vi "Create Private Data for Get Connections Tests.vi"(9 "session":variant, 10 "channel mappings":T1[](array[typedef]), 11 "instrument_type_id":string) -> (3 "data":T2)   [LabVIEW 2020, in "MeasurementServerTests.lvlib"]
uses:
  MeasurementServerTests.lvlib
  Runtime/MeasurementLink Session Management/Session Reservation/Data.ctl
  Runtime/MeasurementLink Session Management/Session Reservation/Session and Driver Info.ctl
  Runtime/MeasurementLink Session Management Client/RPC Messages/ni_measurementlink_sessionmanagement_v1_SessionInformation.ctl
  Runtime/MeasurementLink Session Management Client/RPC Messages/nidevice_grpc_Session.ctl
  Runtime/MeasurementLink Session Management Client/RPC Messages/ni_measurementlink_sessionmanagement_v1_ChannelMapping.ctl
  db59771b-541d-4b59-b44d-886c4f1804c5.vi
  Runtime/MeasurementLink Session Management Client/MeasurementLink Session Management Client.lvlib
  Runtime/MeasurementLink Session Management/Session Reservation/Session Reservation.lvclass
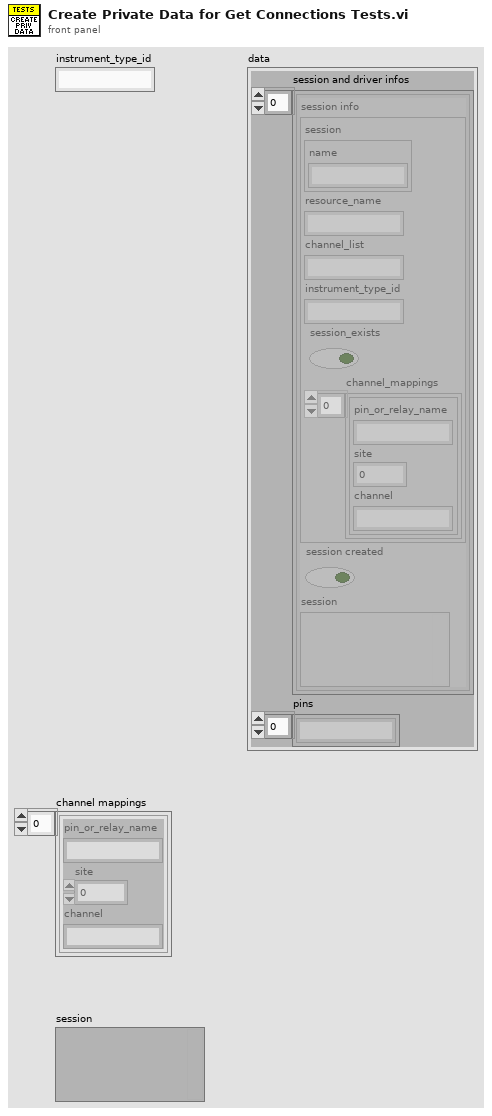
[diagram p1: front panel]
types:
  T1 = typedef "MeasurementLink Session Management Client.lvlib/ni_measurementlink_sessionmanagement_v1_ChannelMapping.ctl" = cluster{"pin_or_relay_name":string, "site":i32, "channel":string}
  T2 = typedef "MeasurementLink Session Management.lvlib/Session Reservation.lvclass/Data.ctl" = cluster{"session and driver infos":T3[], "pins":string[]}
  T3 = typedef "MeasurementLink Session Management.lvlib/Session Reservation.lvclass/Session and Driver Info.ctl" = cluster{"session info":T4, "session created":bool, "session":variant}
  T4 = typedef "MeasurementLink Session Management Client.lvlib/ni_measurementlink_sessionmanagement_v1_SessionInformation.ctl" = cluster{"session":T5, "resource_name":string, "channel_list":string, "instrument_type_id":string, "session_exists":bool, "channel_mappings":T1[]}
  T5 = typedef "MeasurementLink Session Management Client.lvlib/nidevice_grpc_Session.ctl" = cluster{"name":string}
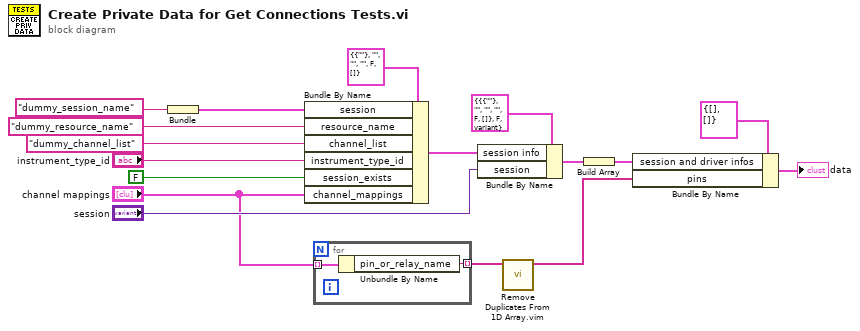
[diagram p0: block diagram]
diagram:
  n1 = Bundle("dummy_session_name") -> (w8:cluster{string})  [unwired: 1 in]
  n2 = Bundle By Name(cluster=T4 {"session"={"name"=""}, "resource_name"="", "channel_list"="", "instrument_type_id"="", "session_exists"=FALSE, "channel_mappings"=[]} ("ni_measurementlink_sessionmanagement_v1_SessionInformation"), "session"=w8, "resource_name"="dummy_resource_name", "channel_list"="dummy_channel_list", "instrument_type_id"="instrument_type_id", "session_exists"=FALSE, "channel_mappings"="channel mappings") -> (w13:T4)
  n3 = for {
    tunnel: "channel mappings" -> [w19] mode=indexing
    tunnel: [w18] -> w1 mode=indexing
    n4 = Unbundle By Name(w19) -> ("pin_or_relay_name"=w18:string)
  }
  n5 = Bundle By Name(cluster=T3 {"session info"={"session"={"name"=""}, "resource_name"="", "channel_list"="", "instrument_type_id"="", "session_exists"=FALSE, "channel_mappings"=[]}, "session created"=FALSE, "session"=variant} ("session and driver info"), "session info"=w13, "session"="session") -> (w14:T3)
  n6 = call "Remove Duplicates From 1D Array.vim"("array"=w1) -> ("array with duplicates removed"=w5:string[])  [unwired: 10 in]
  n7 = Build Array(w14) -> (w16:T3[])
  n8 = Bundle By Name(cluster=T2 {"session and driver infos"=[], "pins"=[]} ("data"), "session and driver infos"=w16, "pins"=w5) -> (→"data":T2)
